vi "Process Messages.vi"(8 "error in (no error)":errorcluster, 11 "Effect Unit in":refnum<class "Effect Unit.lvclass">) -> (0 "error out":errorcluster, 3 "Effect Unit out":refnum<class "Effect Unit.lvclass">)   [LabVIEW 2019, in "Effect Unit.lvclass"]
uses:
  Effect Unit.lvclass
  Effect Unit.lvclass/Effect Unit.ctl
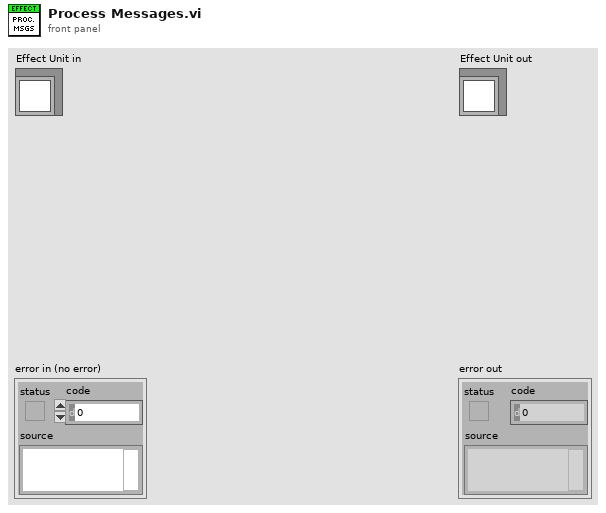
[diagram p1: front panel]
types:
  T1 = typedef "Messaging.lvlib/Message Cluster.ctl" = cluster{"Event":string, "Source":string, "Target":string, "Data":variant}
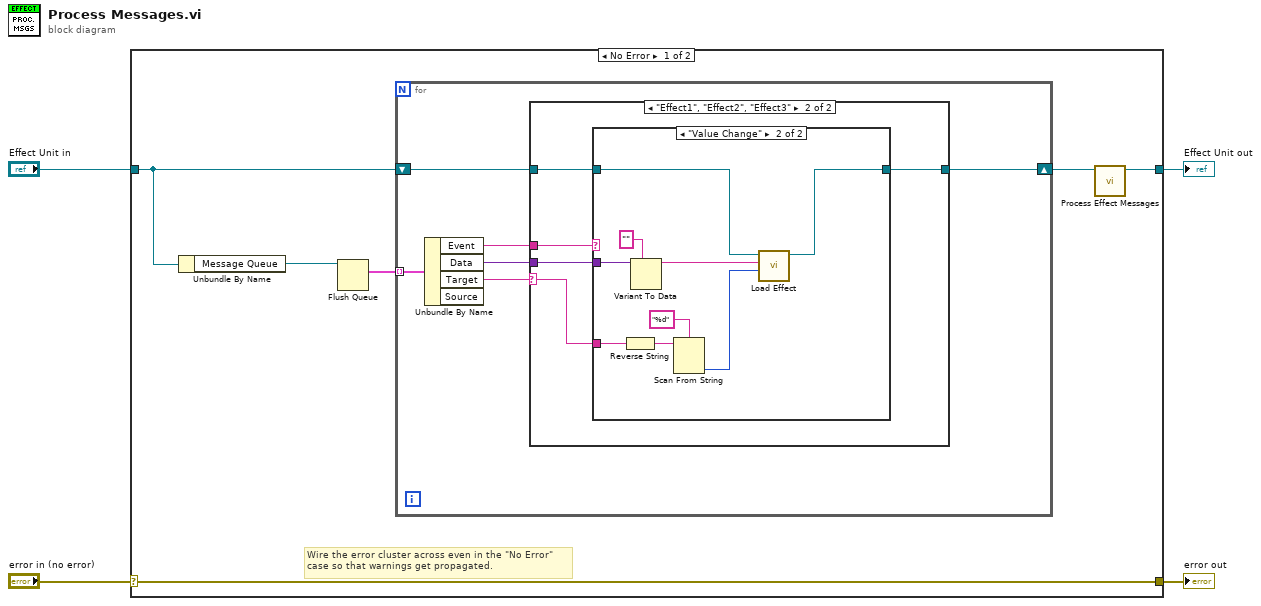
[diagram p0: block diagram]
diagram:
  n1 = case shown="No Error" "error in (no error)" {
    selector: "error in (no error)" -> [w10 w34]
    tunnel: [w10 w34] -> w3
    tunnel: [w9 w33] -> w1
    tunnel: "Effect Unit in" -> [w6 w33]
    frame No Error {
      # "Wire the error cluster across even in the \"No Error\"\ncase so that warnings get propagated."
      n2 = Unbundle By Name(w6) -> ("Message Queue"=w8:refnum<queue>)
      n3 = Flush Queue(queue=w8) -> (remaining elements=w5:T1[])  [unwired: 1 in, 2 out]
      n4 = for {
        shift-right: [w11] -> w7
        shift-left: w6 -> [w12]
        tunnel: w5 -> [w16] mode=indexing
        n5 = Unbundle By Name(w16) -> ("Event"=w13:string, "Data"=w14:variant, "Target"=w15:string)  [unwired: 1 out]
        n6 = case shown="\"Effect1\", \"Effect2\", \"Effect3\"" w15 {
          selector: w15 -> [_ w19]
          tunnel: w14 -> [_ w20]
          tunnel: w13 -> [_ w22]
          tunnel: w12 -> [w17 w21]
          tunnel: [w17 w18] -> w11
          frame Default {
          }
          frame "Effect1", "Effect2", "Effect3" {
            n7 = case shown="\"Value Change\"" w22 {
              tunnel: w21 -> [w23 w32]
              tunnel: w20 -> [_ w31]
              tunnel: w19 -> [_ w28]
              tunnel: [w23 w24] -> w18
              frame Default {
              }
              frame "Value Change" {
                n8 = Reverse String(1:w28) -> (0:w27:string)
                n9 = Variant To Data(type="", Variant=w31) -> (data=w29:string)  [unwired: 1 in, 1 out]
                n10 = Scan From String(format string="%d", input string=w27) -> (output 1=w25:i32)  [unwired: 3 in, 3 out]
                n11 = call "Load Effect.vi"("Effect Slot"=w25, "Effect Name"=w29, "Effect Unit in"=w32) -> ("Effect Unit out"=w24:refnum<class "Effect Unit.lvclass">)  [unwired: 7 in, 1 out]
              }
            }
          }
        }
      }
      n12 = call "Process Effect Messages.vi"("Effect Unit in"=w7) -> ("Effect Unit out"=w9:refnum<class "Effect Unit.lvclass">)  [unwired: 9 in, 1 out]
    }
    frame Error {
    }
  }
  "error out" <- w3
  "Effect Unit out" <- w1
